vi "Save Load Vision.vi"(7 "Name":string, 8 "error in":errorcluster, 10 "Vision Settings (in)":T1={"LED Color"={"Hue"={107.81818389892578, 139.81818389892578}, "Sat"={176.07142857142858, 255.0}, "Val"={40.53571428571429, 255.0}}, "Vision Line"=0.0} {"LED Color"."Hue" scale=0.0..255.0 scale format="%#_3g"}, 11 "Save Load Info (in)":T2) -> (0 "error out":errorcluster, 2 "Vision Settings (out)":T1={"LED Color"={"Hue"={107.81818389892578, 139.81818389892578}, "Sat"={176.07142857142858, 255.0}, "Val"={40.53571428571429, 255.0}}, "Vision Line"=0.0} {"LED Color"."Hue" scale=0.0..255.0 scale format="%#_3g"}, 3 "Save Load Info (out)":T2)   [LabVIEW 2016]
uses:
  Load Save Info.ctl
  <vilib>/Utility/config.llb/Config Data RefNum.ctl
  Vision Data.ctl
  <vilib>/Rock Robotics/Network Tables/NT Write Numeric Array.vi
  <vilib>/Utility/config.llb/Write Key (Double).vi
  <vilib>/Rock Robotics/Network Tables/NT Read Numeric Array.vi
  <vilib>/Utility/config.llb/Read Key (Double).vi
  <vilib>/Utility/config.llb/NI_LVConfig.lvlib
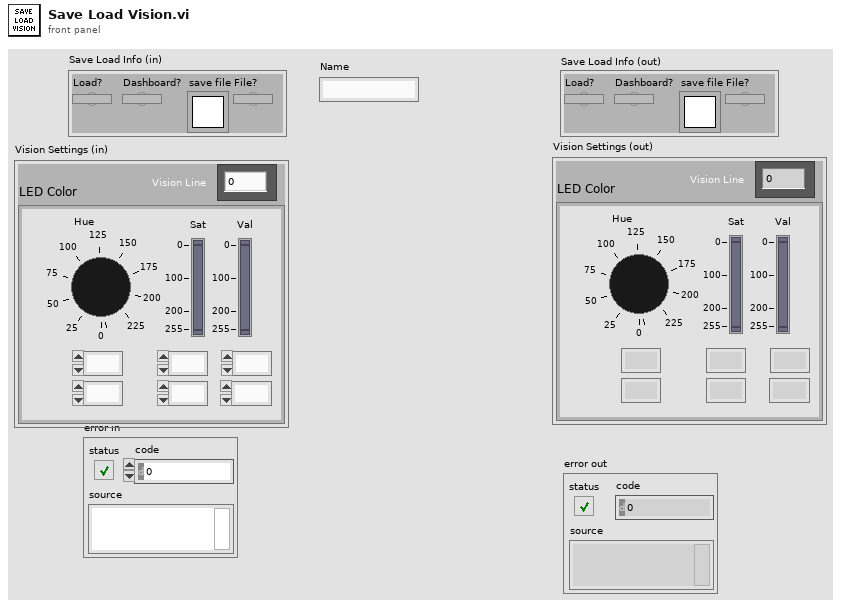
[diagram p1: front panel]
types:
  T1 = typedef "Vision Data.ctl" = cluster{"LED Color":cluster{"Hue":cluster{dbl, dbl}, "Sat":cluster{dbl, dbl}, "Val":cluster{dbl, dbl}}, "Vision Line":dbl}
  T2 = typedef "Load Save Info.ctl" = cluster{"Load?":bool, "Dashboard?":bool, "save file":T3, "File?":bool}
  T3 = typedef "NI_LVConfig.lvlib/Config Data RefNum.ctl" = refnum<k1>
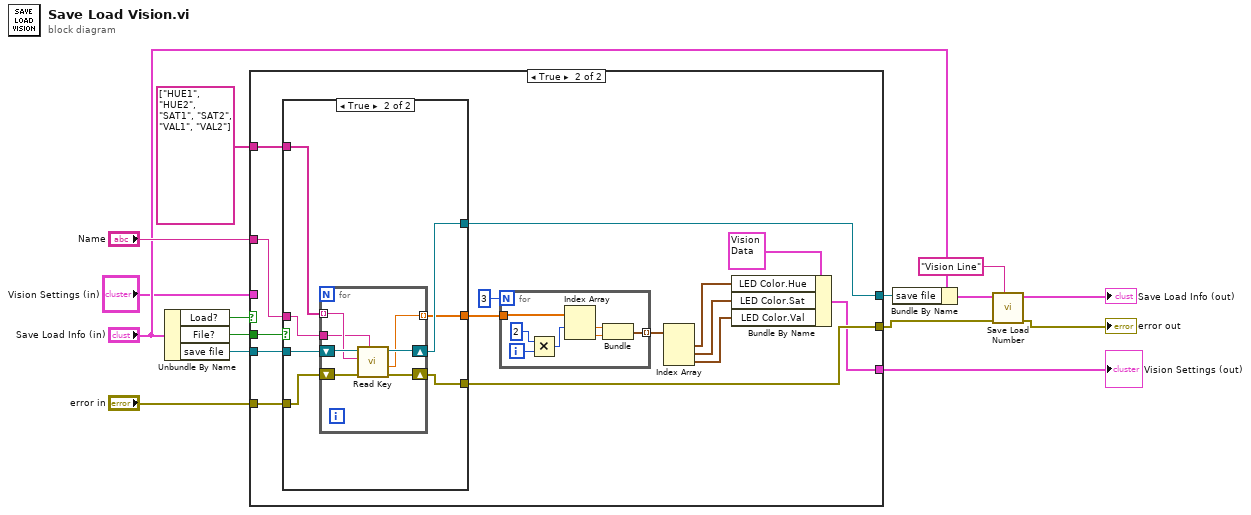
[diagram p0: block diagram]
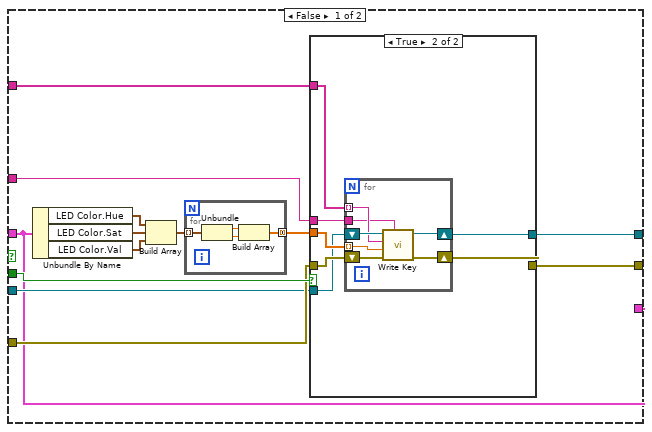
[diagram p2: hidden frame]
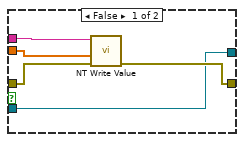
[diagram p3: hidden frame]
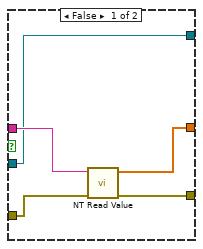
[diagram p4: hidden frame]
diagram:
  n1 = Unbundle By Name("Save Load Info (in)") -> ("Load?"=w15:bool, "File?"=w14:bool, "save file"=w11:T3)
  n2 = case shown="True" w15 {
    tunnel: w14 -> [w28 w66]
    tunnel: "Name" -> [w27 w63]
    tunnel: "Vision Settings (in)" -> [w22 _]
    tunnel: "error in" -> [w26 w65]
    tunnel: w11 -> [w25 w64]
    tunnel: [w24 w61] -> w10
    tunnel: [w23 w62] -> w5
    tunnel: [w22 w60] -> w7
    tunnel: string[] ["HUE1", "HUE2", "SAT1", "SAT2", "VAL1", "VAL2"] -> [w16 w58]
    frame False {
      n3 = Unbundle By Name(w22) -> ("LED Color.Hue"=w21:cluster{dbl, dbl}, "LED Color.Sat"=w20:cluster{dbl, dbl}, "LED Color.Val"=w19:cluster{dbl, dbl})
      n4 = Build Array(w21, w20, w19) -> (w18:cluster{dbl, dbl}[])
      n5 = for {
        tunnel: w18 -> [w32] mode=indexing
        tunnel: [w29] -> w17 mode=concatenating
        n6 = Unbundle(w32) -> (w31:dbl, w30:dbl)
        n7 = Build Array(w31, w30) -> (w29:dbl[])
      }
      n8 = case shown="True" w28 {
        tunnel: w27 -> [w37 w43]
        tunnel: w17 -> [w36 w42]
        tunnel: w26 -> [w35 w44]
        tunnel: [w34 w41] -> w23
        tunnel: w25 -> [w33 w40]
        tunnel: [w33 w39] -> w24
        tunnel: w16 -> [_ w38]
        frame False {
          n9 = call-poly <vilib>:"NT Write Value.vi"("error in"=w35, "Numeric Array"=w36, "Name"=w37) -> ("error out"=w34:errorcluster)  [unwired: 8 in]
        }
        frame True {
          n10 = for {
            tunnel: w43 -> [w47]
            tunnel: w38 -> [w48] mode=indexing
            shift-right: [w49] -> w41
            shift-left: w44 -> [w50]
            shift-right: [w46] -> w39
            shift-left: w40 -> [w51]
            tunnel: w42 -> [w45] mode=indexing
            n11 = call-poly <vilib>:"Write Key.vi"("section"=w47, "error in (no error)"=w50, "value"=w45, "key"=w48, "refnum"=w51) -> ("error out"=w49:errorcluster, "refnum out"=w46:T3)  [unwired: 4 in, 1 out]
          }
        }
      }
    }
    frame True {
      n12 = case shown="True" w66 {
        tunnel: w65 -> [w78 w85]
        tunnel: w64 -> [w74 w84]
        tunnel: w63 -> [w76 w83]
        tunnel: [w77 w82] -> w62
        tunnel: [w74 w81] -> w61
        tunnel: [w75 w80] -> w56
        tunnel: w58 -> [_ w79]
        frame False {
          n13 = call-poly <vilib>:"NT Read Value.vi"("error in"=w78, "Name"=w76) -> ("error out"=w77:errorcluster, "Numeric Array"=w75:dbl[])  [unwired: 8 in]
        }
        frame True {
          n14 = for {
            tunnel: w83 -> [w88]
            tunnel: w79 -> [w89] mode=indexing
            shift-right: [w90] -> w82
            shift-left: w85 -> [w91]
            shift-right: [w87] -> w81
            shift-left: w84 -> [w92]
            tunnel: [w86] -> w80 mode=indexing
            n15 = call-poly <vilib>:"Read Key.vi"("section"=w88, "error in (no error)"=w91, "key"=w89, "refnum"=w92) -> ("error out"=w90:errorcluster, "value"=w86:dbl, "refnum out"=w87:T3)  [unwired: 4 in, 1 out]
          }
        }
      }
      n16 = for {
        N: 3 -> [_]
        tunnel: w56 -> [w71]
        tunnel: [w67] -> w55 mode=indexing
        i -> [w73]
        n17 = Multiply(x=2, y=w73) -> (x*y=w70:i32)
        n18 = Index Array(array=w71, index #1=w70) -> (element #1=w68:dbl, element #2=w69:dbl)  [unwired: 1 in]
        n19 = Bundle("value"=w68, "value"=w69) -> (w67:cluster{"value":dbl, "value":dbl})  [unwired: 1 in]
      }
      n20 = Index Array(array=w55) -> (element #1=w54:cluster{"value":dbl, "value":dbl}, element #2=w53:cluster{"value":dbl, "value":dbl}, element #3=w52:cluster{"value":dbl, "value":dbl})  [unwired: 3 in]
      n21 = Bundle By Name(cluster=T1 {"LED Color"={"Hue"={107.81818389892578, 139.81818389892578}, "Sat"={176.07142857142858, 255.0}, "Val"={40.53571428571429, 255.0}}, "Vision Line"=0.0} ("Vision Settings (in) 2"), "LED Color.Hue"=w54, "LED Color.Sat"=w53, "LED Color.Val"=w52) -> (w60:T1)
    }
  }
  "Vision Settings (out)" <- w7
  n22 = Bundle By Name(cluster="Save Load Info (in)", "save file"=w10) -> (w3:T2)
  n23 = call "Save Load Number.vi"("Name"="Vision Line", "error in"=w5, "Save Load Info (in)"=w3) -> ("error out"=→"error out":errorcluster, "Save Load Info (out)"=→"Save Load Info (out)":T2)  [unwired: 6 in, 1 out]
